vi "LKIF_SetProgramNo.vi"(8 "error in (no error)":errorcluster {"code" format="%x"}, 11 "ProgramNo":i32) -> (0 "error out":errorcluster {"code" format="%x"})   [LabVIEW 8.6, in "Keyence LK-G3000.lvlib"]
uses:
  Keyence LK-G3000.lvlib
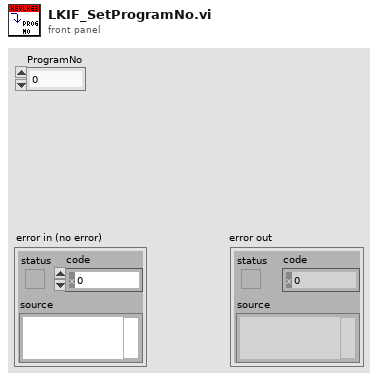
[diagram p1: front panel]
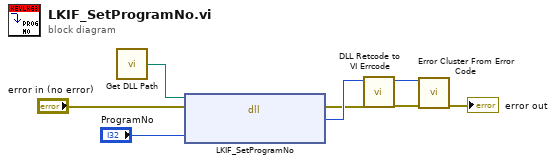
[diagram p0: block diagram]
diagram:
  n1 = call "Get DLL Path.vi"() -> ("DLL Path"=w1:path)  [unwired: 1 in]
  n2 = dll-call lib="C:/Program Files/National Instruments/LabVIEW 2011/instr.lib/Keyence LK-G3000/LkIF.dll" fn="LKIF_SetProgramNo"(path in=w1, error in="error in (no error)", "ProgramNo"="ProgramNo") -> (error out=w2:errorcluster, "RC"=w3:i32)  [unwired: 2 in, 1 out]
  n3 = call "DLL Retcode to VI Errcode.vi"("error in (no error)"=w2, "DLL Retcode"=w3) -> ("error out"=w8:errorcluster, "VI Errcode"=w7:i32)  [unwired: 8 in]
  n4 = call <vilib>:"Error Cluster From Error Code.vi"("error in (no error)"=w8, "error code (0)"=w7) -> ("error out"=→"error out":errorcluster)  [unwired: 7 in]
